vi "UnInit.vi"(1 "error in (no error)":errorcluster, 2 "IGxFactory":refnum<k24>) -> (0 "error out":errorcluster)   [LabVIEW 2013, in "GxLVlib.lvlib"]
uses:
  GxLVlib.lvlib
  F:/GxILibrary/Labview/trunk/private/dev/src/C#/x86/GxLVLib/dll/GxIAPINET.dll
  private/dev/src/C#/x86/GxLVLib/dll/GxIAPINET.dll
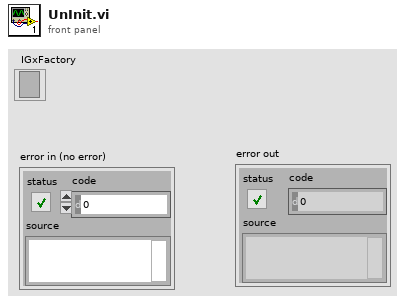
[diagram p1: front panel]
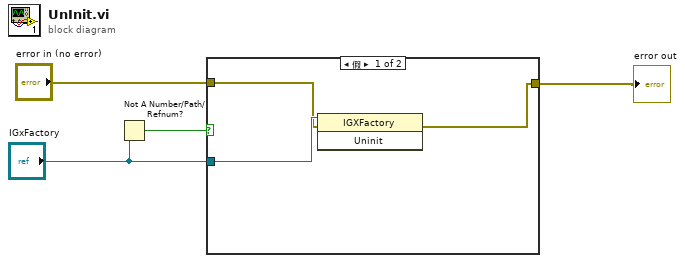
[diagram p0: block diagram]
diagram:
  n1 = Not A Number/Path/Refnum?(number/path/refnum="IGxFactory") -> (NaN/Path/Refnum?=w4:bool)
  n2 = case shown="假" w4 {
    tunnel: "error in (no error)" -> [w6 w8]
    tunnel: [w5 w8] -> w2
    tunnel: "IGxFactory" -> [w7 _]
    frame False {
      n3 = invoke class="IGXFactory" method="Uninit"(reference=w7, error in=w6) -> (error out=w5:errorcluster)  [unwired: 1 in, 2 out]
    }
    frame True {
    }
  }
  "error out" <- w2
